vi "pthread_condattr_getclock.vi"(8 "error in (no error)":errorcluster, 11 "cond attr ptr in":u64) -> (0 "error out":errorcluster, 2 "clock id":T1=enum."Monotonic", 3 "cond attr ptr out":u64)   [LabVIEW 2013, in "Linux RT IPC.POSIX Threads.lvlib" / "POSIX Thread Object.lvclass"]
uses:
  POSIX Thread Object.lvclass
  <vilib>/NI/NI Linux RT Utilities/Controls/Public/C Enums/clockid_t.ctl
  Controls/pthread functions.ctl
  <vilib>/NI/NI Linux RT Utilities/Linux RT Utilities.lvlib
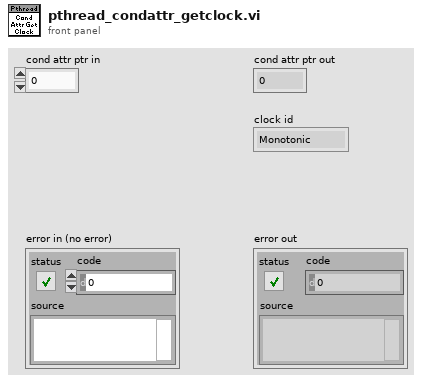
[diagram p1: front panel]
types:
  T1 = typedef "Linux RT Utilities.lvlib/clockid_t.ctl" = enum16{"Realtime", "Monotonic"}
  T2 = typedef "Linux RT IPC.POSIX Threads.lvlib/POSIX Thread Object.lvclass/pthread functions.ctl" = enum16{"unspecified", "pthread_condattr_init", "pthread_condattr_destroy", "pthread_condattr_getclock", "pthread_condattr_setclock", "pthread_condattr_getpshared", "pthread_condattr_setpshared", "pthread_cond_init", "pthread_cond_destroy", "pthread_cond_broadcast", "pthread_cond_signal", "pthread_cond_timedwait", "pthread_cond_wait", "pthread_mutexattr_init", "pthread_mutexattr_destroy", "pthread_mutexattr_getprioceiling", "pthread_mutexattr_setprioceiling", "pthread_mutexattr_getprotocol", "pthread_mutexattr_setprotocol", "pthread_mutexattr_getpshared", "pthread_mutexattr_setpshared", "pthread_mutexattr_gettype", "pthread_mutexattr_settype", "pthread_mutex_init", "pthread_mutex_destroy", "pthread_mutex_getprioceiling", "pthread_mutex_setprioceiling", "pthread_mutex_lock", "pthread_mutex_timedlock", "pthread_mutex_trylock", "pthread_mutex_unlock", "sem_destroy", "sem_getvalue", "sem_init", "sem_post", "sem_timedwait", "sem_trywait", "sem_wait", "barrier_init", "barrier_destroy", "barrier_wait", "barrierattr_init", "barrierattr_destroy", "barrierattr_getpshared", "barrierattr_setpshared"}
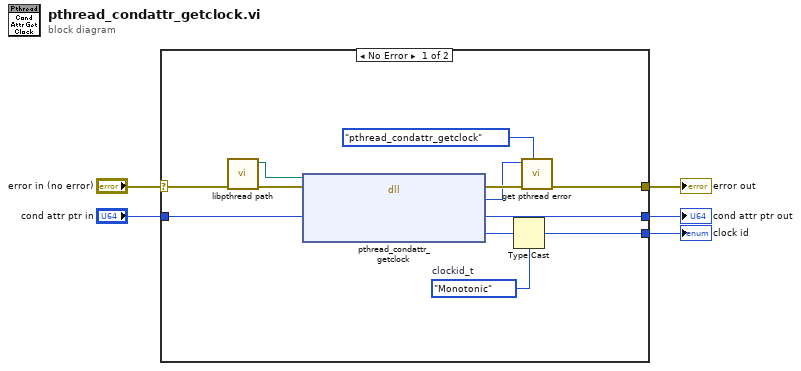
[diagram p0: block diagram]
diagram:
  n1 = case shown="No Error" "error in (no error)" {
    selector: "error in (no error)" -> [w17 w19]
    tunnel: "cond attr ptr in" -> [w16 w18]
    tunnel: [w15 w19] -> w3
    tunnel: [w14 _] -> w2
    tunnel: [w13 w18] -> w1
    frame No Error {
      w6 = clockid_t."Monotonic"  # clockid_t
      n2 = call "libpthread path.vi"("error in (no error)"=w17) -> ("error out"=w11:errorcluster, "path to libpthread"=w12:path)  [unwired: 9 in]
      n3 = dll-call lib="?" fn="pthread_condattr_getclock"(path in=w12, error in=w11, "cond attr"=w16) -> (error out=w10:errorcluster, "errno"=w9:i32, "cond attr"=w13:u64, "clock_id"=w7:i32)  [unwired: 2 in, 1 out]
      n4 = Type Cast(type=w6, x=w7) -> (*(type *) &x=w14:T1)
      n5 = call "get pthread error.vi"("function"=pthread_functions."pthread_condattr_getclock", "error in (no error)"=w10, "errno"=w9) -> ("error out"=w15:errorcluster)  [unwired: 8 in]
    }
    frame Error {
    }
  }
  "error out" <- w3
  "clock id" <- w2
  "cond attr ptr out" <- w1
